vi "Curtin1_SoundCardCorrection.vi"(10 "Settings":T1={"Name of test"="", "Date"=timestamp(0 s since 1904-01-01), "Location"="", "Template"="", "Soundcard"="", "resolution"=0, "Sampling rate"=0, "Ch1 Gain "=0.0, "Ch2 Gain"=0.0, "Sample time (s)"=0.0, "Pre-trigger (s)"=0.0, "Hammer Threshold"=0.0, "Positions"=0, "Taps/Position"=0, "Set Names"="", "Freq resolution"=0.0, "Hammer cutoff"=0.0, "Mic cutoff"=0.0, "Double bounce "=0.0, "Hammer Cal"=0.0, "dB Offset"=0.0, "Accel Cal"=0.0, "Vibrometer Cal"=0.0, "Mic Cal"=0.0, "Output"=0, "Voltage Cal"=0.0, "Vibrometer Port"="ASRL27::INSTR", "Range"=4, "High Pass"=2, "Bandwidth"=4, "X Range"=[], "Y Range"=[], "dB Spread"=0.0, "Trigger"=0, "Ch_1"=25, "Ch_2"=25, "flip?"=FALSE, "60Hz"=FALSE, "Time offset"=0.0, "Piezo Cal"=1.0, "Default Notes"="", "Tom"=FALSE} {"Ch_2" min=1 step=1; "Ch_1" min=1 max=100 step=1; "Trigger" items=["Hammer (force)", "Self-tap", "Spacebar"]; "Bandwidth" items=["1 kHz"=1, "5 kHz"=5, "10 kHz"=10, "25 kHz"=25, "50 kHz"=50, "100 kHz"=100]; "High Pass" items=["Off", "13 Hz", "104 Hz"]; "Range" items=["10 mm/s"=1, "20 mm/s"=2, "50 mm/s"=5, "100 mm/s"=10, "200 mm/s"=20, "500 mm/s"=50, "1 m/s"=100, "2 m/s"=200]; "Output" items=["Accelerometer", "Speed (from acceleration)", "Microphone", "Vibrometer", "Piezo"]; "Voltage Cal" format="%#_13g"; "Ch2 Gain" format="%#_13g"; "Ch1 Gain" format="%#_13g"; "Double bounce" min=0.0; "Mic cutoff" min=0.0 format="%#_4g"; "Hammer cutoff" min=0.0 format="%#_4g"; "Freq resolution" min=0.0; "Pre-trigger (s)" format="%#_13g"; "Date" format="%<%H:%M\n%d/%m/%y>T"; "resolution" items=["16 bit"=16, "24 bit"=24, "32 bit"=32]; "Sampling rate" items=["22050 samp/s"=22050, "44100 samp/s"=44100, "48000 samp/s"=48000]}, 11 "Buffer in":waveform(dbl)[](graph)) -> (0 "Microphone":waveform(dbl)[](graph), 1 "Hammer":waveform(dbl)[](graph), 2 "SPL":dbl, 3 "Volts Out":waveform(dbl)[](graph), 4 "Converted":dbl[](array[numeric]), 5 "rms calibrated value":dbl format="%0.2f")   [LabVIEW 2022 SP3]
uses:
  <vilib>/Analysis/NI_AALPro.lvlib
  <vilib>/Analysis/5stat.llb/RMS (DBL).vi
  PreferencesControl.ctl
panel:
  # "Buffer is microphone, hammer"
  # "Hz"
  # "dB"
  # "dB"
  # "sec"
  # "sec"
  # "mV/Pa"
  # "mV/m/s2"
  # "mV/mm/s"
  # "V/N"
  # "sec"
  # "sec"
  # "mV/N"
  # "%"
  # "%"
  # "sec"
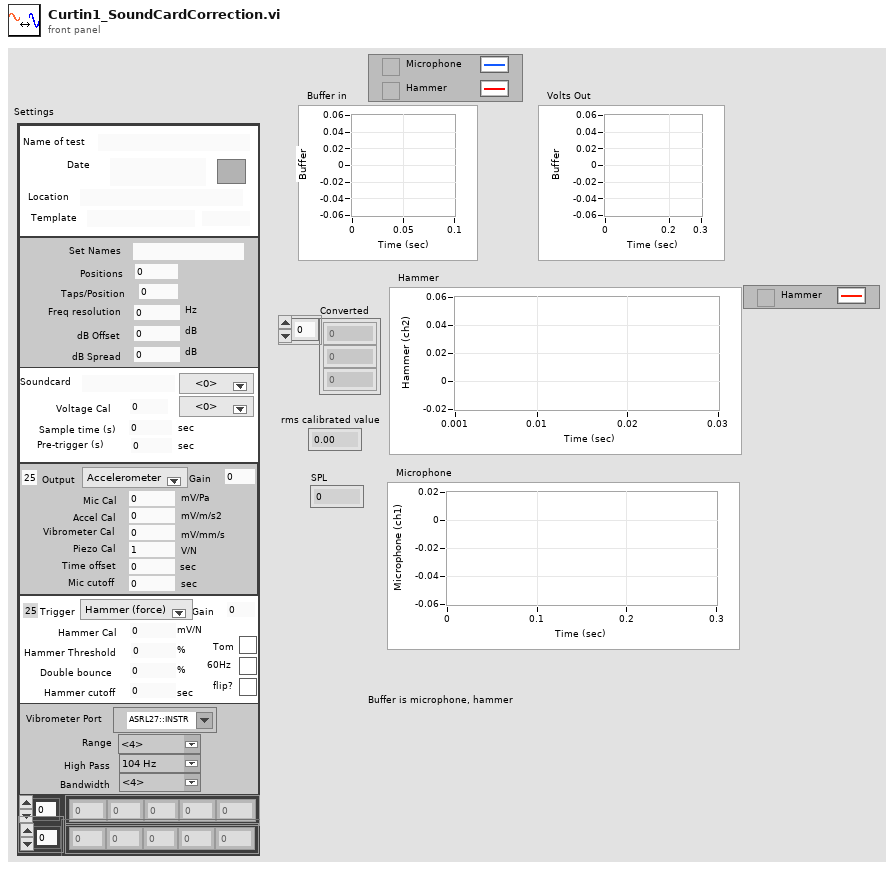
[diagram p1: front panel]
types:
  T1 = typedef "PreferencesControl.ctl" = cluster{"Name of test":string, "Date":timestamp, "Location":string, "Template":string, "Soundcard":string, "resolution":u16, "Sampling rate":u16, "Ch1 Gain ":dbl, "Ch2 Gain":dbl, "Sample time (s)":dbl, "Pre-trigger (s)":dbl, "Hammer Threshold":dbl, "Positions":i16, "Taps/Position":i16, "Set Names":string, "Freq resolution":dbl, "Hammer cutoff":dbl, "Mic cutoff":dbl, "Double bounce ":dbl, "Hammer Cal":dbl, "dB Offset":dbl, "Accel Cal":dbl, "Vibrometer Cal":dbl, "Mic Cal":dbl, "Output":u16, "Voltage Cal":dbl, "Vibrometer Port":refnum<visa-resource-name>, "Range":u16, "High Pass":u16, "Bandwidth":u16, "X Range":cluster{"Minimum":dbl, "Maximum":dbl, "Increment":dbl, "Minor Increment":dbl, "Start":dbl}[], "Y Range":cluster{"Minimum":dbl, "Maximum":dbl, "Increment":dbl, "Minor Increment":dbl, "Start":dbl}[], "dB Spread":dbl, "Trigger":u16, "Ch_1":u8, "Ch_2":u8, "flip?":bool, "60Hz":bool, "Time offset":dbl, "Piezo Cal":dbl, "Default Notes":string, "Tom":bool}
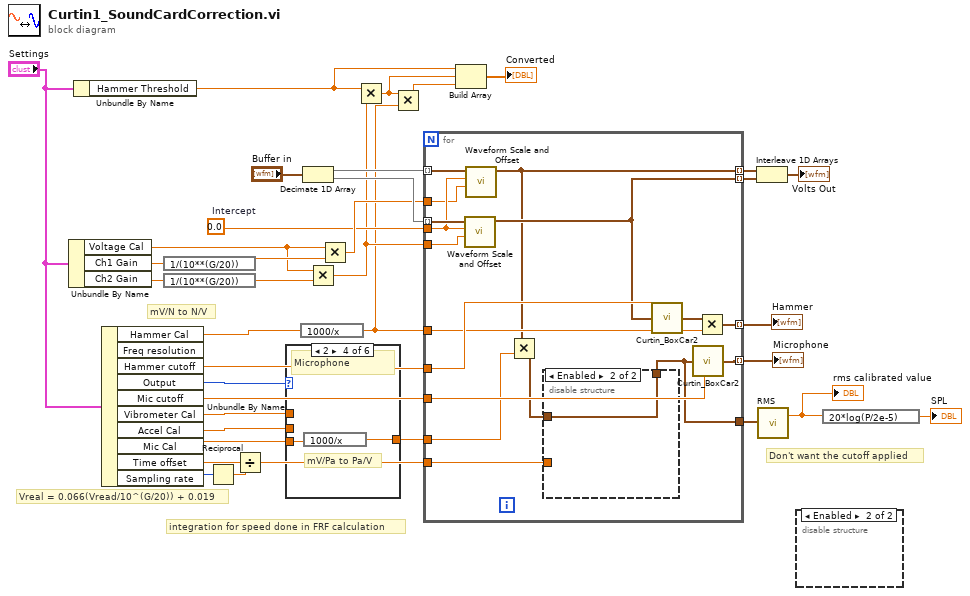
[diagram p0: block diagram]
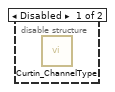
[diagram p2: hidden frame]
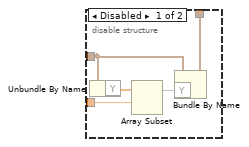
[diagram p3: hidden frame]
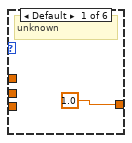
[diagram p4: hidden frame]
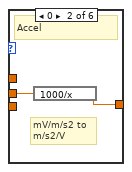
[diagram p5: hidden frame]
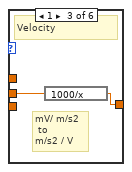
[diagram p6: hidden frame]
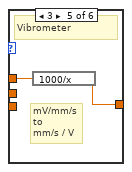
[diagram p7: hidden frame]
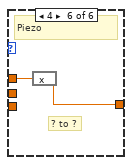
[diagram p8: hidden frame]
diagram:
  w16 = 0.0  # Intercept
  # "integration for speed done in FRF calculation"
  # "Don't want the cutoff applied"
  # "mV/N to N/V"
  # "Vreal = 0.066(Vread/10^(G/20)) + 0.019"
  n1 = Unbundle By Name("Settings") -> ("Voltage Cal"=w20:dbl, "Ch1 Gain"=w24:dbl, "Ch2 Gain"=w21:dbl)
  n2 = Unbundle By Name("Settings") -> ("Hammer Threshold"=w10:dbl)
  n3 = Unbundle By Name("Settings") -> ("Hammer Cal"=w5:dbl, "Hammer cutoff"=w35:dbl, "Output"=w33:u16, "Mic cutoff"=w34:dbl, "Vibrometer Cal"=w37:dbl, "Accel Cal"=w36:dbl, "Mic Cal"=w6:dbl, "Time offset"=w2:dbl, "Sampling rate"=w4:u16)  [unwired: 1 out]
  n4 = expression code="1/(10**(G/20))"(w24) -> (w31:dbl)
  n5 = expression code="1/(10**(G/20))"(w21) -> (w22:dbl)
  n6 = Reciprocal(x=w4) -> (1/x=w3:dbl)
  n7 = Divide(x=w2, y=w3) -> (x/y=w1:dbl)
  n8 = case shown="2" w33 {
    tunnel: [1.0 ("Vibrometer Cal") w39 w41 w43 w45 w47] -> w32
    tunnel: w37 -> [_ _ _ _ w46 w48]
    tunnel: w36 -> [_ w40 w42 _ _ _]
    tunnel: w6 -> [_ _ _ w44 _ _]
    frame Default {
      # "unknown"
    }
    frame 0 {
      # "mV/m/s2 to \nm/s2/V"
      # "Accel"
      n9 = expression code="1000/x"(w40) -> (w39:dbl)
    }
    frame 1 {
      # "mV/ m/s2 \n to\nm/s2 / V"
      # "Velocity"
      n10 = expression code="1000/x"(w42) -> (w41:dbl)
    }
    frame 2 {
      # "mV/Pa to Pa/V"
      # "Microphone"
      n11 = expression code="1000/x"(w44) -> (w43:dbl)
    }
    frame 3 {
      # "mV/mm/s\nto\nmm/s / V"
      # "Vibrometer"
      n12 = expression code="1000/x"(w46) -> (w45:dbl)
    }
    frame 4 {
      # "? to ?"
      # "Piezo"
      n13 = expression code="x"(w48) -> (w47:dbl)
    }
  }
  n14 = expression code="1000/x"(w5) -> (w12:dbl)
  n15 = Decimate 1D Array("Buffer in") -> (w29:waveform(dbl)[], w28:waveform(dbl)[])
  n16 = Multiply(x=w20, y=w22) -> (x*y=w13:dbl)
  n17 = Multiply(x=w20, y=w31) -> (x*y=w23:dbl)
  n18 = Multiply(x=w10, y=w13) -> (x*y=w9:dbl)
  n19 = Multiply(x=w9, y=w12) -> (x*y=w8:dbl)
  n20 = for {
    tunnel: w35 -> [w64]
    tunnel: w34 -> [w63]
    tunnel: w12 -> [w62]
    tunnel: w32 -> [w54]
    tunnel: [w52] -> w15 mode=indexing
    tunnel: [w61] -> w19 mode=indexing
    tunnel: w29 -> [w60] mode=indexing
    tunnel: w28 -> [w59] mode=indexing
    tunnel: [w53] -> w27 mode=indexing
    tunnel: [w55] -> w26 mode=indexing
    tunnel: w16 -> [w58]
    tunnel: w23 -> [w57]
    tunnel: w13 -> [w56]
    tunnel: [w50] -> w14
    tunnel: w1 -> [w49]
    n21 = call <vilib>:"Waveform Scale and Offset.vi"("scale"=w56, "offset"=w58, "waveform in"=w59) -> ("waveform out"=w55:waveform(dbl))  [unwired: 7 in, 1 out]
    n22 = call <vilib>:"Waveform Scale and Offset.vi"("scale"=w57, "offset"=w58, "waveform in"=w60) -> ("waveform out"=w53:waveform(dbl))  [unwired: 7 in, 1 out]
    n23 = Multiply(x=w53, y=w54) -> (x*y=w51:waveform(dbl))
    n24 = disable-structure shown="Enabled" {
      disable-tunnel: w51 -> [w70 w71]
      disable-tunnel: [w69 w71] -> w50
      disable-tunnel: w49 -> [w66 _]
      frame Disabled {
        n25 = Unbundle By Name(w70) -> ("Y"=w68:dbl[])
        n26 = Array Subset(array=w68, index=w66) -> (w67:dbl[])  [unwired: 1 in]
        n27 = Bundle By Name(cluster=w70, "Y"=w67) -> (w69:waveform(dbl))
      }
      frame Enabled {
      }
    }
    n28 = call "Curtin_BoxCar2.vi"("Original Data"=w55, "Cutoff (sec)"=w64) -> ("Cutoff Data"=w65:waveform(dbl))  [unwired: 1 in]
    n29 = call "Curtin_BoxCar2.vi"("Original Data"=w50, "Cutoff (sec)"=w63) -> ("Cutoff Data"=w52:waveform(dbl))  [unwired: 1 in]
    n30 = Multiply(x=w65, y=w62) -> (x*y=w61:waveform(dbl))
  }
  "Hammer" <- w19
  "Microphone" <- w15
  n31 = Build Array(w10, w9, w8) -> (→"Converted":dbl[])
  n32 = Interleave 1D Arrays(w27, w26) -> (→"Volts Out":waveform(dbl)[])
  n33 = call-poly <vilib>:"RMS.vi"("X"=w14) -> ("rms value"=w18:dbl)  [unwired: 1 out]
  "rms calibrated value" <- w18
  n34 = disable-structure shown="Enabled" {
    frame Disabled {
      n35 = call "Curtin_ChannelType.vi"() -> ()  [unwired: 3 in, 1 out]
    }
    frame Enabled {
    }
  }
  n36 = expression code="20*log(P/2e-5)"(w18) -> (→"SPL":dbl)
